vi "AlignPosition2.vi"(6 "Chip Orientation":i32, 7 "Steps Per micron":dbl, 9 "Position 1":i32[](array[numeric]), 10 "Microsites":refnum<k24>, 11 "Boolean in":refnum<vi>) -> (2 "Array":dbl[](array[numeric]), 3 "Numeric":dbl)   [LabVIEW 2020]
uses:
  C:/Users/User/Desktop/Automation/NextVersion/DXFViewer/LabviewDXFViewer/LabviewDXFViewer/bin/Release/LabviewDXFViewer.exe
  LabviewDXFViewer/bin/Release/LabviewDXFViewer.exe
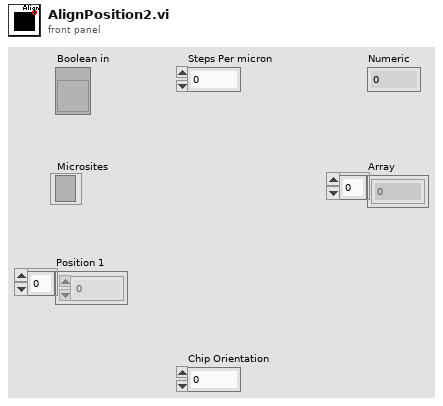
[diagram p1: front panel]
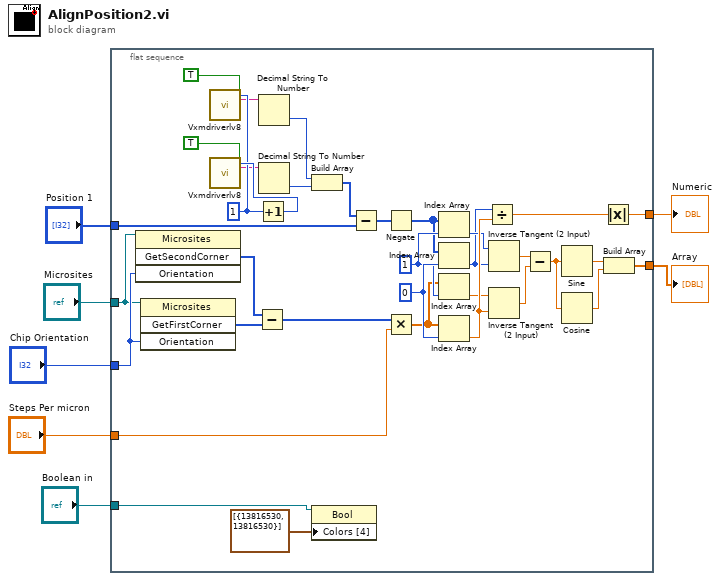
[diagram p0: block diagram]
diagram:
  n1 = flat-sequence {
    tunnel: "Microsites" -> [w24]
    tunnel: "Chip Orientation" -> [w25]
    tunnel: [w12] -> w3
    tunnel: [w11] -> w4
    tunnel: "Position 1" -> [w10]
    tunnel: "Boolean in" -> [w9]
    tunnel: "Steps Per micron" -> [w8]
    frame #0 {
      w31 = 1 ("index")
      w33 = 0 ("index")
      w41 = 1 ("Motor\nNumber")
      n2 = invoke class="Microsites" method="GetSecondCorner"(reference=w24, "Orientation"=w25) -> ("GetSecondCorner"=w29:i32[])  [unwired: 2 in, 3 out]
      n3 = invoke class="Microsites" method="GetFirstCorner"(reference=w24, "Orientation"=w25) -> ("GetFirstCorner"=w22:i32[])  [unwired: 2 in, 3 out]
      n4 = call "Vxmdriverlv8.Vi"("Get\nMotor\nPosition"=TRUE ("Get\nMotor\nPosition"), "Motor\nNumber"=w41) -> ("Motor Position"=w38:string)  [unwired: 20 in, 5 out]
      n5 = Subtract(x=w29, y=w22) -> (x-y=w23:i32[])
      n6 = Increment(x=w41) -> (x+1=w42:i32)
      n7 = call "Vxmdriverlv8.Vi"("Get\nMotor\nPosition"=TRUE ("Get\nMotor\nPosition"), "Motor\nNumber"=w42) -> ("Motor Position"=w37:string)  [unwired: 20 in, 5 out]
      n8 = Decimal String To Number(string=w38) -> (number=w35:i32)  [unwired: 2 in, 1 out]
      n9 = Decimal String To Number(string=w37) -> (number=w36:i32)  [unwired: 2 in, 1 out]
      n10 = Build Array(w35, w36) -> (w34:i32[])
      n11 = property class="Bool"(reference=w9, "Colors [4]"=cluster{u32, u32}[] [{13816530, 13816530}]) -> ()  [unwired: 1 in, 2 out]
      n12 = Subtract(x=w34, y=w10) -> (x-y=w30:i32[])
      n13 = Negate(x=w30) -> (-x=w20:i32[])
      n14 = Multiply(x=w23, y=w8) -> (x*y=w21:dbl[])
      n15 = Index Array(array=w20, index=w31) -> (element=w17:i32)
      n16 = Index Array(array=w20, index=w33) -> (element=w16:i32)
      n17 = Index Array(array=w21, index=w31) -> (element=w18:dbl)
      n18 = Index Array(array=w21, index=w33) -> (element=w19:dbl)
      n19 = Divide(x=w16, y=w19) -> (x/y=w32:dbl)
      n20 = Inverse Tangent (2 Input)(1:w16, 2:w17) -> (0:w28:dbl)
      n21 = Inverse Tangent (2 Input)(1:w19, 2:w18) -> (0:w14:dbl)
      n22 = Subtract(x=w28, y=w14) -> (x-y=w15:dbl)
      n23 = Sine(x=w15) -> (sin(x)=w27:dbl)
      n24 = Cosine(x=w15) -> (cos(x)=w26:dbl)
      n25 = Absolute Value(x=w32) -> (abs(x)=w12:dbl)
      n26 = Build Array(w27, w26) -> (w11:dbl[])
    }
  }
  "Array" <- w4
  "Numeric" <- w3
